vi "表换线提示.vi"(8 "error in (no error)":errorcluster caption="错误输入（无错误）", 10 "接线状态":i32, 11 "Fluke 8808A 输入":refnum<class "Fluke 8808A.lvclass">) -> (0 "error out":errorcluster caption="错误输出", 3 "Fluke 8808A 输出":refnum<class "Fluke 8808A.lvclass">)   [LabVIEW 2020, in "Fluke 8808A.lvlib" / "Fluke 8808A.lvclass"]
uses:
  Fluke 8808A.lvclass
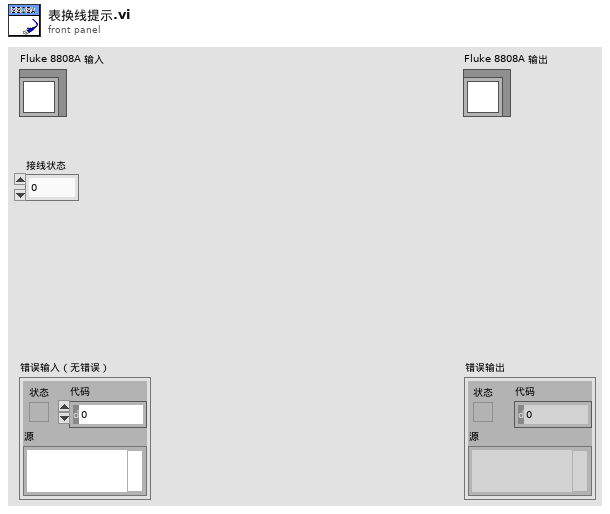
[diagram p1: front panel]
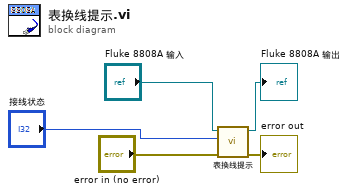
[diagram p0: block diagram]
diagram:
  n1 = call-parent "表换线提示.vi"("error in (no error)"="error in (no error)", "接线状态"="接线状态", "数字多用表接口 输入"="Fluke 8808A 输入") -> ("error out"=→"error out":errorcluster, "数字多用表接口 输出"=→"Fluke 8808A 输出":refnum<class "Fluke 8808A.lvclass">)  [unwired: 7 in]
